vi "InterfaceNeuro.vi"() -> ()   [LabVIEW 2017]
uses:
  <vilib>/Analysis/1siggen.llb/Ramp Pattern by Samples.vi
  <vilib>/Utility/file.llb/Read Delimited Spreadsheet (DBL).vi
  <vilib>/Analysis/NI_AALBase.lvlib
panel:
  in  "stop 2":bool
  in  "Tiempo de\nestímulo":dbl
  in  "Comenzar \nprueba":bool
  in  "Cantidad de \ncuadros":dbl
  out "Amplitud\nP100 2":dbl
  out "N75 2":dbl
  out "P100 2":dbl
  out "N145 2":dbl
  out "Latencia  2":dbl
  out "Amplitud\nP100":dbl
  out "N75":dbl
  out "P100":dbl
  out "N145":dbl
  out "Latencia":dbl
  out "Resultado de las pruebas 2":cluster{"first row":dbl[], "Ramp Pattern":dbl[]}(graph)
  in  "stop":bool
  out "Resultado de las pruebas":cluster{"first row":dbl[], "Ramp Pattern":dbl[]}(graph)
  # "Resultados promedio"
  # "Resultados promedio"
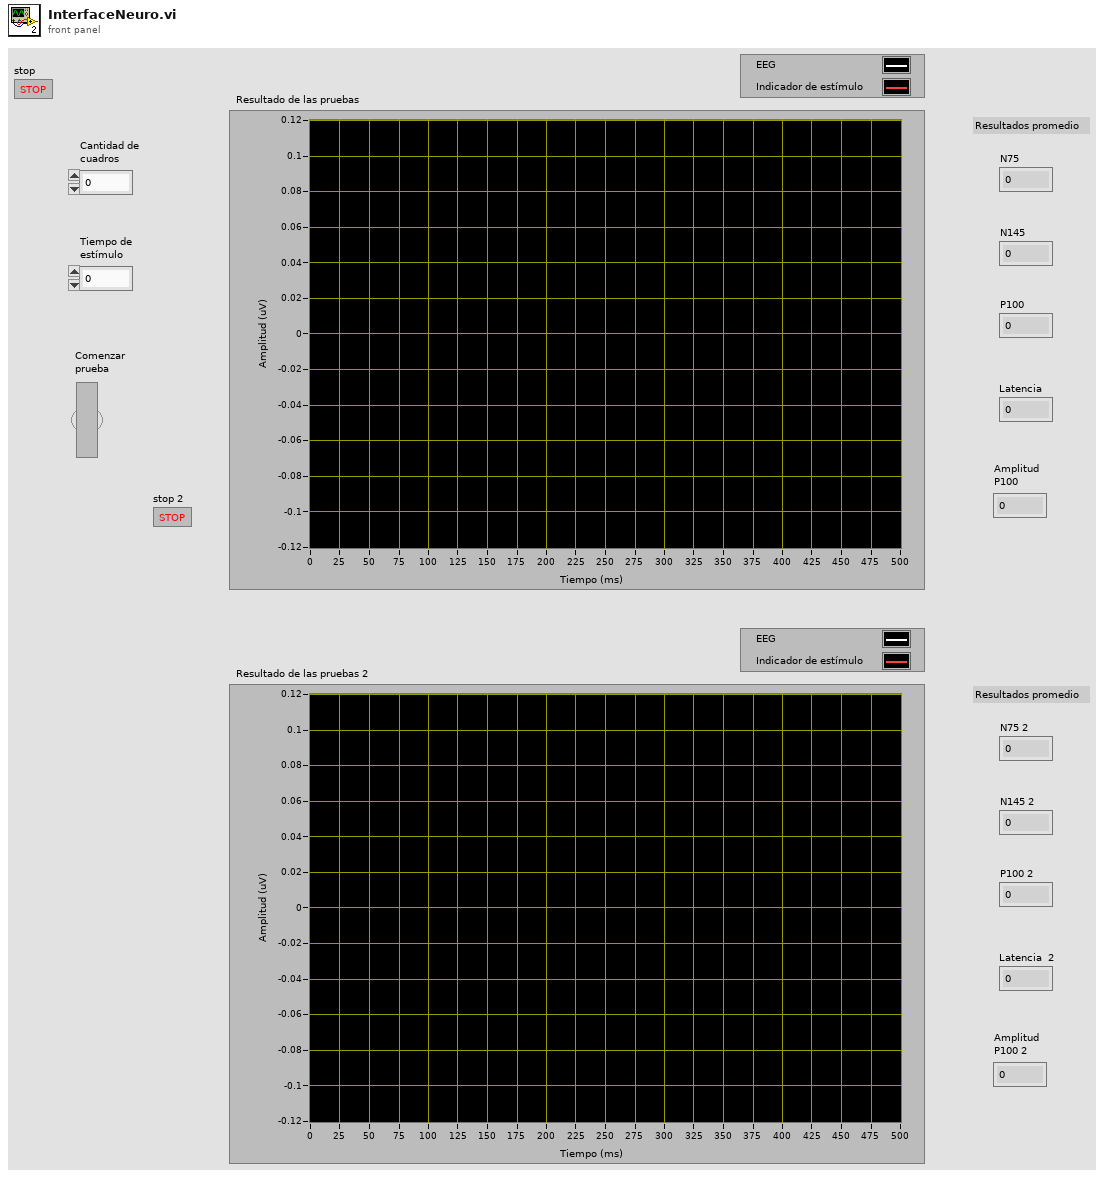
[diagram p1: front panel]
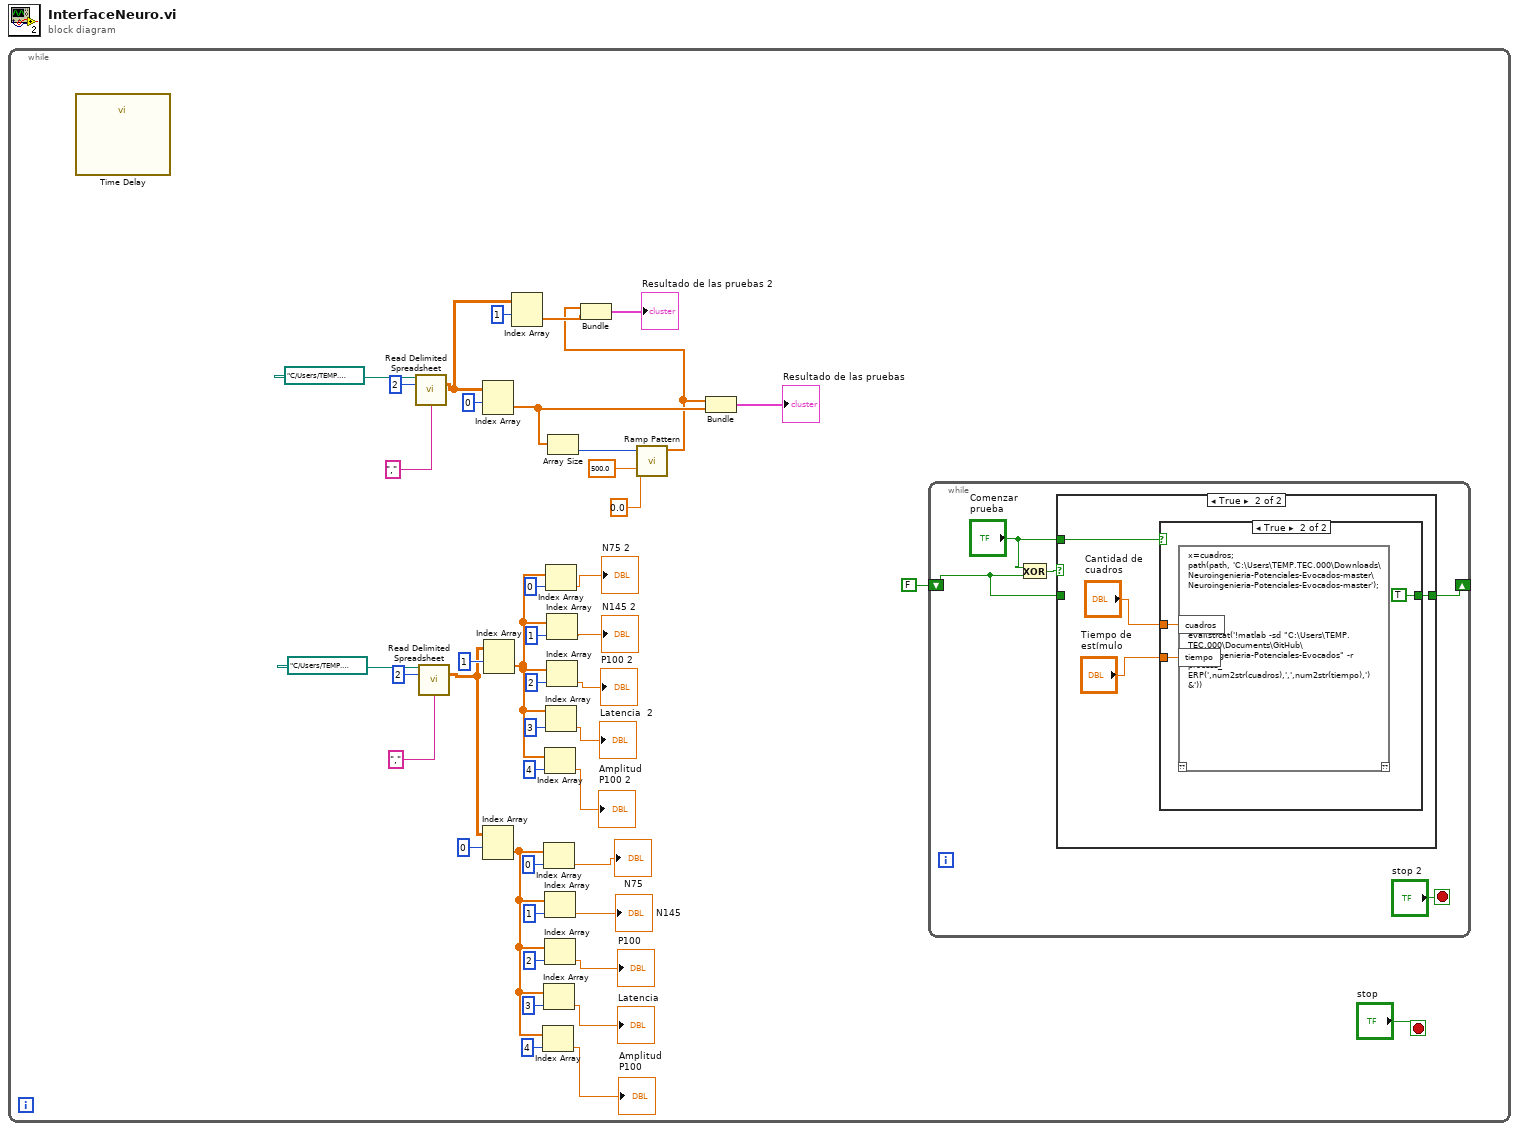
[diagram p0: block diagram]
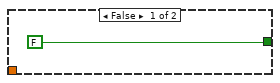
[diagram p3: hidden frame]
diagram:
  n1 = while {
    stop <- "stop" stop-if-true
    n2 = call "Time Delay"() -> ()  [unwired: 11 in, 1 out]
    n3 = call-poly <vilib>:"Read Delimited Spreadsheet.vi"("file path (dialog if empty)"=path "C:/Users/TEMP.TEC.000/Documents/GitHub/Neuroingenieria-Potenciales-Evocados/prueba.csv", "number of rows (all:-1)"=2, "delimiter (\\t)"="," ("delimiter (\\t)")) -> ("all rows"=w33:dbl[][])  [unwired: 7 in, 5 out]
    n4 = call-poly <vilib>:"Read Delimited Spreadsheet.vi"("file path (dialog if empty)"=path "C:/Users/TEMP.TEC.000/Documents/GitHub/Neuroingenieria-Potenciales-Evocados/resultados.csv", "number of rows (all:-1)"=2, "delimiter (\\t)"="," ("delimiter (\\t)")) -> ("all rows"=w24:dbl[][])  [unwired: 7 in, 5 out]
    n5 = Index Array(array=w33, index (row)=0) -> (element=w35:dbl[])  [unwired: 1 in]
    n6 = Index Array(array=w24, index (row)=0) -> (element=w18:dbl[])  [unwired: 1 in]
    n7 = Index Array(array=w24, index (row)=1) -> (element=w12:dbl[])  [unwired: 1 in]
    n8 = Index Array(array=w33, index (row)=1) -> (element=w32:dbl[])  [unwired: 1 in]
    n9 = Index Array(array=w18, index=4) -> (element=→"Amplitud\nP100":dbl)
    n10 = Index Array(array=w18, index=0) -> (element=→"N75":dbl)
    n11 = Index Array(array=w18, index=3) -> (element=→"Latencia":dbl)
    n12 = Index Array(array=w12, index=4) -> (element=→"Amplitud\nP100 2":dbl)
    n13 = Index Array(array=w18, index=1) -> (element=→"N145":dbl)
    n14 = Index Array(array=w18, index=2) -> (element=→"P100":dbl)
    n15 = Index Array(array=w12, index=0) -> (element=→"N75 2":dbl)
    n16 = Index Array(array=w12, index=3) -> (element=→"Latencia  2":dbl)
    n17 = Index Array(array=w12, index=1) -> (element=→"N145 2":dbl)
    n18 = Index Array(array=w12, index=2) -> (element=→"P100 2":dbl)
    n19 = Array Size(array=w35) -> (size(s)=w37:i32)
    n20 = call-poly <vilib>:"Ramp Pattern.vi"("start"=0.0, "end"=500.0, "samples"=w37) -> ("Ramp Pattern"=w31:dbl[])  [unwired: 7 in, 1 out]
    n21 = Bundle("Ramp Pattern"=w31, "all rows"=w32) -> (→"Resultado de las pruebas 2":cluster{"Ramp Pattern":dbl[], "all rows":dbl[]})  [unwired: 1 in]
    n22 = Bundle("Ramp Pattern"=w31, "all rows"=w35) -> (→"Resultado de las pruebas":cluster{"Ramp Pattern":dbl[], "all rows":dbl[]})  [unwired: 1 in]
    n23 = while {
      shift-right: [w49] -> _
      shift-left: FALSE -> [w47]
      stop <- "stop 2" stop-if-true
      n24 = Exclusive Or(1:w47, 2:"Comenzar \nprueba") -> (0:w48:bool)
      n25 = case shown="True" w48 {
        tunnel: [w50 w54] -> w49
        tunnel: "Comenzar \nprueba" -> [_ w53]
        tunnel: w47 -> [w50 _]
        frame False {
        }
        frame True {
          n26 = case shown="True" w53 {
            tunnel: [FALSE TRUE] -> w54
            tunnel: "Cantidad de \ncuadros" -> [_ w57]
            tunnel: "Tiempo de\nestímulo" -> [_ w56]
            frame False {
            }
            frame True {
              n27 = script code="x=cuadros;\npath(path, 'C:\\Users\\TEMP.TEC.000\\Downloads\\Neuroingenieria-Potenciales-Evocados-master\\Neuroingenieria-Potenciales-Evocados-master');\n\n\n\n\neval(strcat('!matlab -sd \"C:\\Users\\TEMP.TEC.000\\Documents\\GitHub\\Neuroingenieria-Potenciales-Evocados\" -r process_ERP(',num2str(cuadros),',',num2str(tiempo),') &'))"("cuadros"=w57, "tiempo"=w56) -> ()  [unwired: 1 in, 1 out]
            }
          }
        }
      }
    }
  }
